vi "replace all vi icon of message maker with good one.vi"() -> ()   [LabVIEW 2014]
panel:
  out "class name":string
  out "Class Hierarchy":string[][](array[string])
  out "Array":path[](array[path])
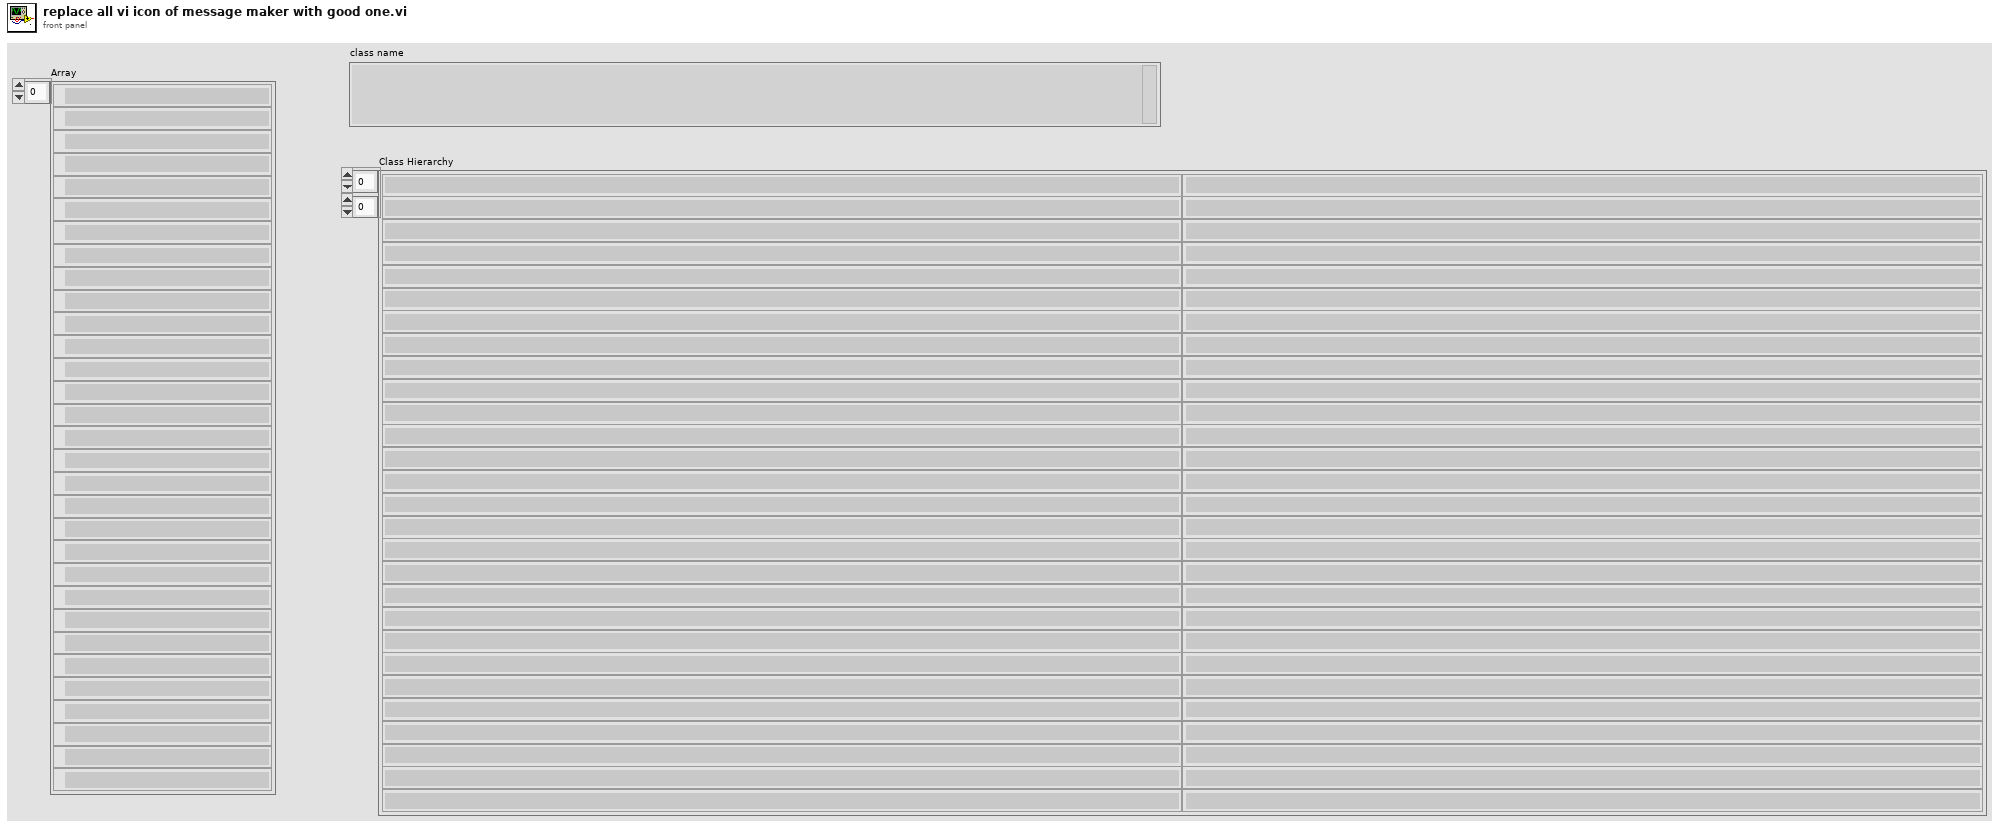
[diagram p1: front panel]
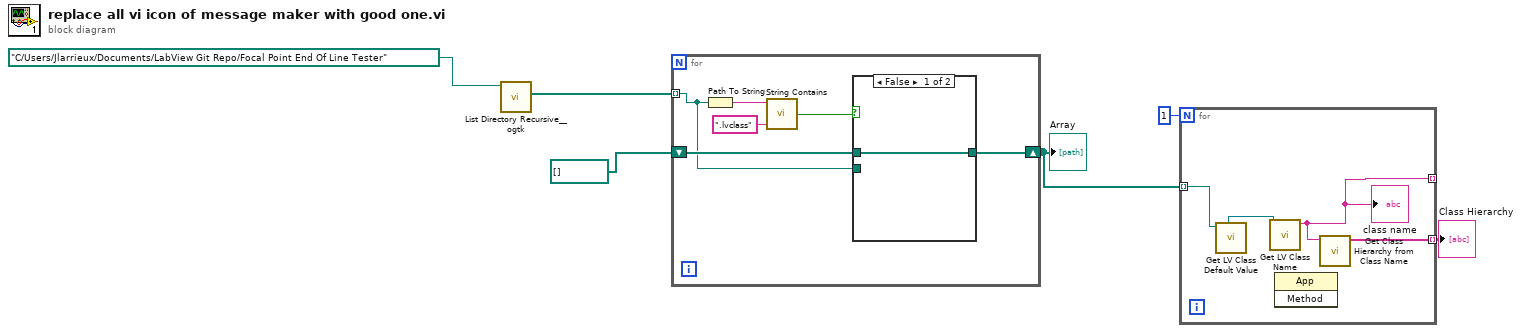
[diagram p0: block diagram]
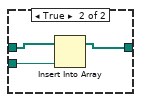
[diagram p2: hidden frame]
diagram:
  n1 = call <userlib>:"List Directory Recursive__ogtk.vi"("Path"=path "C:/Users/Jlarrieux/Documents/LabView Git Repo/Focal Point End Of Line Tester") -> ("file paths"=w5:path[])  [unwired: 7 in, 3 out]
  n2 = for {
    tunnel: w5 -> [w7] mode=indexing
    shift-right: [w8] -> w3
    shift-left: path[] [] -> [w9]
    n3 = Path To String(path=w7) -> (string=w12:string)
    n4 = call "String Contains.vi"("Regular expression"=".lvclass", "Input String"=w12) -> ("Boolean"=w10:bool)  [unwired: 3 in]
    n5 = case shown="False" w10 {
      tunnel: w9 -> [w13 w16]
      tunnel: [w13 w14] -> w8
      tunnel: w7 -> [_ w15]
      frame False {
      }
      frame True {
        n6 = Insert Into Array(array=w16, new element=w15) -> (w14:path[])  [unwired: 1 in]
      }
    }
  }
  "Array" <- w3
  n7 = for {
    N: 1 -> [_]
    tunnel: w3 -> [w20] mode=indexing
    tunnel: [w19] -> w1 mode=indexing
    tunnel: [w18] -> _ mode=indexing
    n8 = call <vilib>:"Get LV Class Default Value.vi"("class path"=w20) -> ("object"=w17:refnum<class>)  [unwired: 9 in, 1 out]
    n9 = call <vilib>:"Get LV Class Name.vi"("object"=w17) -> ("class name"=w18:string)  [unwired: 9 in, 1 out]
    "class name" <- w18
    n10 = invoke class="App" method=#-1() -> ()  [unwired: 3 in, 3 out]
    n11 = call <vilib>:"Get Class Hierarchy from Class Name.vi"("Class Name"=w18) -> ("Class Hierarchy"=w19:string[])  [unwired: 9 in, 1 out]
  }
  "Class Hierarchy" <- w1
